vi "Separate Taps and Weights.vi"(7 "Filter Size":i32, 10 "Array in":fxp<+/-,24,8>[](array[numeric]) format="%.19g") -> (2 "Array out":fxp<+/-,24,8>[][](array[numeric]) format="%.19g")   [LabVIEW 2016]
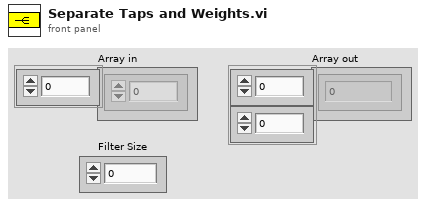
[diagram p1: front panel]
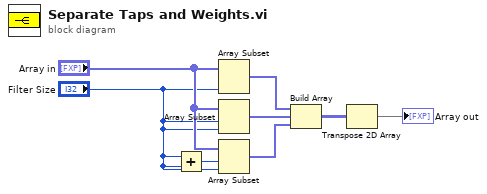
[diagram p0: block diagram]
diagram:
  n1 = Add(x="Filter Size", y="Filter Size") -> (x+y=w6:i32)
  n2 = Array Subset(array="Array in", length="Filter Size") -> (w4:fxp<+/-,24,8>[])  [unwired: 1 in]
  n3 = Array Subset(array="Array in", index="Filter Size", length="Filter Size") -> (w5:fxp<+/-,24,8>[])
  n4 = Array Subset(array="Array in", index=w6, length="Filter Size") -> (w3:fxp<+/-,24,8>[])
  n5 = Build Array(w4, w5, w3) -> (w2:fxp<+/-,24,8>[][])
  n6 = Transpose 2D Array(2D array=w2) -> (transposed array=→"Array out":fxp<+/-,24,8>[][])
